vi "Create Pulse Waveform File.vi"(6 "error in":errorcluster, 9 "filename":path=path "C:/5-01-003 Active Electrode Min Max/Waveform Sq Pos Pulse.dat") -> (0 "error out":errorcluster, 3 "Waveform":waveform(dbl)(graph)={"t0"=timestamp(3473168073.631 s since 1904-01-01), "dt"=0.001, "Y"=array[1000 elements], "attributes"=variant("Average Size"=variant(dbl 15.0), "NSamp"=variant(dbl 400000.0), "Resistance (ohms)"=variant(dbl 500.0), "Samp Freq (MHz)"=variant(dbl 100.0), "dt (us)"=variant(dbl 0.01))})   [LabVIEW 2010]
uses:
  <vilib>/Waveform/WDTFileIO.llb/ Write Waveform to File.vi
panel:
  in  "Stimulus":T1={"Positive Polarity"=FALSE, "amplitude"=2.0, "pulse width"=400, "interphase delay"=400, "rise time"=500, "fall time"=500} {"amplitude" format="%.3f"}
  in  "nelem (1000)":i32=1000
  in  "offset":dbl=0.5 format="%.3f"
  in  "append file (F)":bool
  in  "parameters":waveform(dbl)={"t0"=timestamp(3473168073.631 s since 1904-01-01), "dt"=0.001, "Y"=[], "attributes"=variant("Average Size"=variant(dbl 15.0), "NSamp"=variant(dbl 400000.0), "Resistance (ohms)"=variant(dbl 500.0), "Samp Freq (MHz)"=variant(dbl 100.0), "dt (us)"=variant(dbl 0.01))}
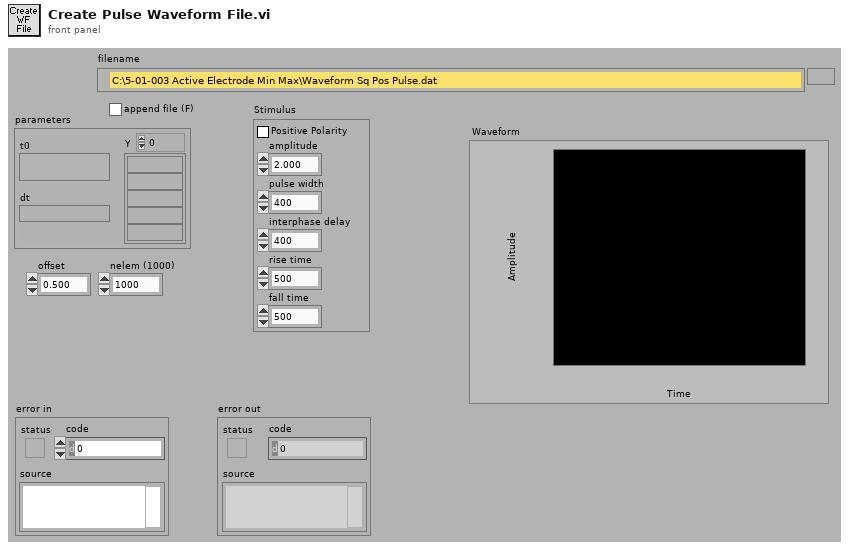
[diagram p1: front panel]
types:
  T1 = cluster{"Positive Polarity":bool, "amplitude":dbl, "pulse width":i32, "interphase delay":i32, "rise time":i32, "fall time":i32}
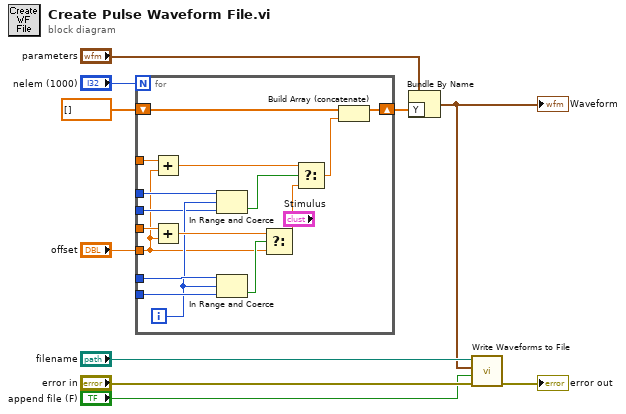
[diagram p0: block diagram]
diagram:
  n1 = for {
    N: "nelem (1000)" -> [_]
    tunnel: [w30] -> w10
    shift-right: [w32] -> w7
    shift-left: dbl[] [] -> [w31]
    tunnel: "offset" -> [w21]
    tunnel: [w29] -> w5
    tunnel: [w26] -> w4
    tunnel: [w24] -> w3
    tunnel: [w23] -> w2
    tunnel: [w20] -> w1
    i -> [w25]
    n2 = Add(x=w20, y=w21) -> (x+y=w19:dbl)
    n3 = Add(x=w26, y=w21) -> (x+y=w27:dbl)
    n4 = In Range and Coerce(upper limit=w23, x=w25, lower limit=w24) -> (In Range?=w18:bool)  [unwired: 1 out]
    n5 = In Range and Coerce(upper limit=w29, x=w25, lower limit=w30) -> (In Range?=w28:bool)  [unwired: 1 out]
    n6 = Select(t=w27, s=w28, f=w21) -> (s? t:f=w22:dbl)
    n7 = Select(t=w19, s=w18, f=w22) -> (s? t:f=w17:dbl)
    n8 = Build Array (concatenate) "Build Array"(w31, w17) -> (w32:dbl[])
  }
  n9 = Bundle By Name(cluster="parameters", "Y"=w7) -> (w12:waveform(dbl))
  "Waveform" <- w12
  n10 = call-poly <vilib>:"Write Waveforms to File.vi"("error in (no error)"="error in", "append to file? (new file:F)"="append file (F)", "waveform"=w12, "file path (dialog if empty)"="filename") -> ("error out"=→"error out":errorcluster)  [unwired: 6 in, 1 out]
